vi "PNG Loader.vi"() -> ()   [LabVIEW 2020, in "App.lvclass"]
uses:
  App/App.lvclass
panel:
  in  "Path":path=path "C:/dev/LabVIEW/Good Company Calc/Data/Images/Battery Stack.png"
  out "new picture":picture
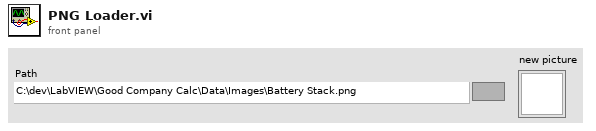
[diagram p1: front panel]
types:
  T1 = typedef "imagedata.ctl" = cluster{"image type":i32, "image depth":i32, "image":u8[], "mask":u8[], "colors":u32[], "Rectangle":cluster{"left":i16, "top":i16, "right":i16, "bottom":i16}}
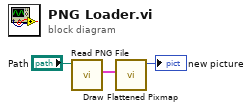
[diagram p0: block diagram]
diagram:
  n1 = call <vilib>:"Read PNG File.vi"("path to PNG file"="Path") -> ("image data"=w2:T1)  [unwired: 8 in, 2 out]
  n2 = call <vilib>:"Draw Flattened Pixmap.vi"("image data"=w2) -> ("new picture"=→"new picture":picture)  [unwired: 8 in]
